vi "DrawOverlayImage.vi"(0 "reference":refnum<class "PackageNode.lvclass">, 1 "graphics":refnum<class "Graphics.lvclass">, 5 "error in (no error)":errorcluster) -> (14 "reference out":refnum<class "PackageNode.lvclass">, 15 "HotSpots":T1[](array[typedef]) {"HotSpot"."y" format="%.2f"; "HotSpot"."x" format="%.2f"}, 19 "error out":errorcluster)   [LabVIEW 2020, in "PackageNode.lvclass"]
doc: "Abstract draw"
uses:
  <resource>/Framework/Providers/Open_GDS/UML/PackageNode_class/PackageNode.lvclass
  C:/Program Files (x86)/National Instruments/LabVIEW 2020/resource/Framework/Providers/Open_GDS/UML/RectangularNode_class/RectangularNode.lvclass
  C:/Program Files (x86)/National Instruments/LabVIEW 2020/resource/Framework/Providers/Open_GDS/UML/AbstractNode_class/AbstractNode.lvclass
  <resource>/Framework/Providers/Open_GDS/UML/Graphics_class/Graphics.lvclass
  <resource>/Framework/Providers/Open_GDS/UML/UMLEditor/UMLEditor_HotSpotData.ctl
  <resource>/Framework/Providers/Open_GDS/UML/AbstractNode_class/AbstractNode.lvclass
  <resource>/Framework/Providers/Open_GDS/UML/General/Point/Point Point2D.ctl
  <resource>/Framework/Providers/Open_GDS/UML/UMLEditor/UMLEditor_HotSpotType.ctl
  <vilib>/picture/picture.llb/imagedata.ctl
  <resource>/Framework/Providers/Open_GDS/UML/RectangularNode_class/RectangularNode.lvclass
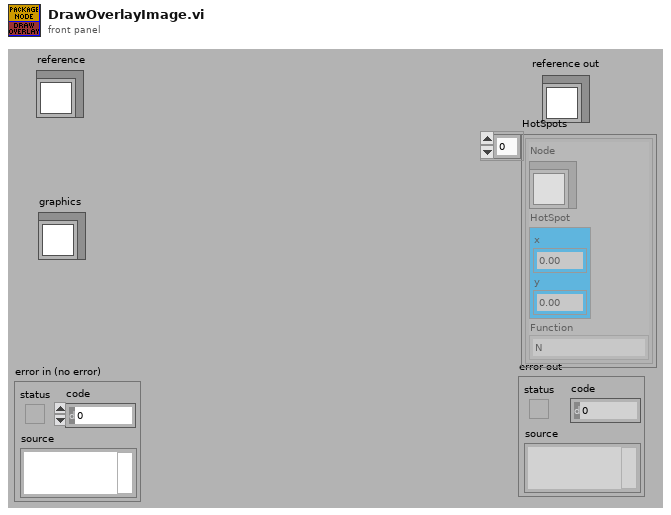
[diagram p1: front panel]
types:
  T1 = typedef "UMLEditor_HotSpotData.ctl" = cluster{"Node":refnum<class "AbstractNode.lvclass">, "HotSpot":T2, "Function":T3}
  T2 = typedef "Point Point2D.ctl" = cluster{"x":dbl, "y":dbl}
  T3 = typedef "UMLEditor_HotSpotType.ctl" = enum16{"N", "NE", "E", "SE", "S", "SW", "W", "NW", "Expand", "Collaps"}
  T4 = typedef "imagedata.ctl" = cluster{"image type":i32, "image depth":i32, "image":u8[], "mask":u8[], "colors":u32[], "Rectangle":cluster{"left":i16, "top":i16, "right":i16, "bottom":i16}}
  T5 = typedef "PackageNode.lvclass/ObjectAttributes.ctl" = cluster{"name":string, "contents":refnum<class "MultiLineString.lvclass">, "DEFAULT_TOP_WIDTH":i32, "DEFAULT_TOP_HEIGHT":i32, "DEFAULT_WIDTH":i32, "DEFAULT_HEIGHT":i32, "NAME_GAP":i32, "XGAP":i32, "YGAP":i32, "Collapsed":bool, "Note color":u32, "Justification":u16}
  T6 = typedef "RectangularNode.lvclass/ObjectAttributes.ctl" = cluster{"bounds":T7}
  T7 = typedef "Rectangle Rectangle2D.ctl" = cluster{"x":dbl, "y":dbl, "width":dbl, "height":dbl}
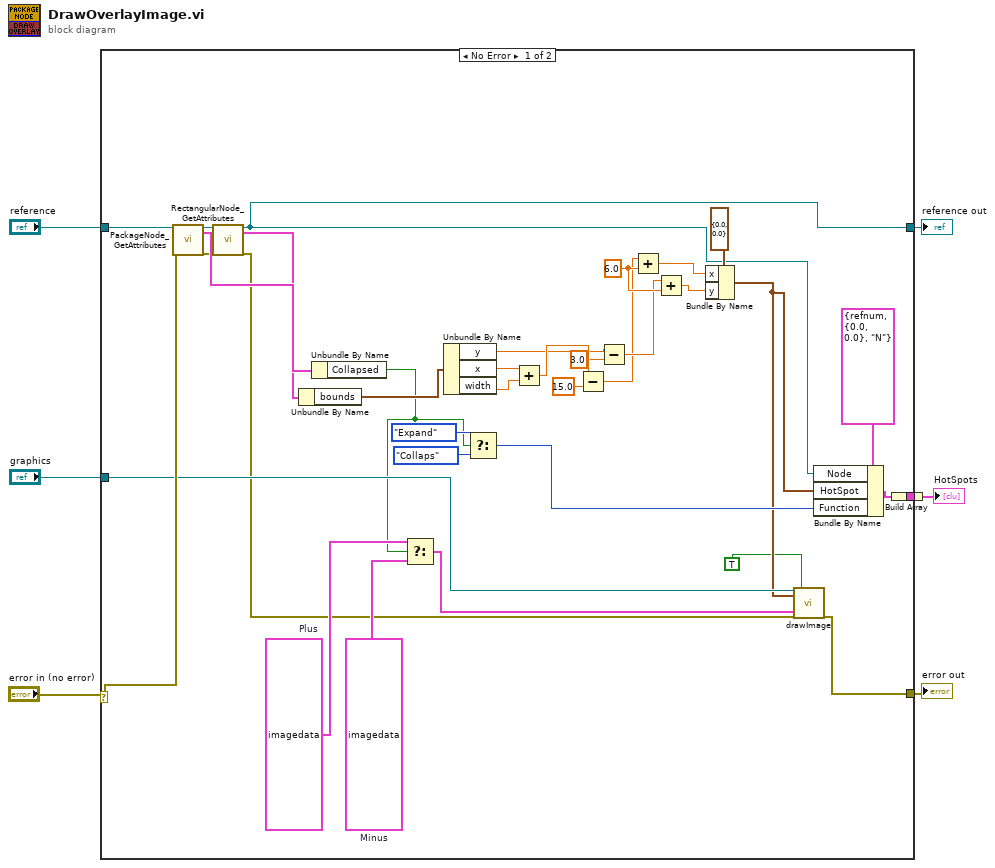
[diagram p0: block diagram]
diagram:
  n1 = case shown="No Error" "error in (no error)" {
    selector: "error in (no error)" -> [w40 w42]
    tunnel: "reference" -> [w41 w43]
    tunnel: [w39 w42] -> w5
    tunnel: [w8 w43] -> w4
    tunnel: "graphics" -> [w31 _]
    tunnel: [w25 _] -> w1
    frame No Error {
      w22 = 6.0 ("y")
      w29 = T4 {"image type"=0, "image depth"=24, "image"=[255, 255, 255, 255, 255, 255, 219, 227, 245, 189, 201, 232, 163, 178, 221, 155, 173, 221, 154, 171, 218, 154, 169, 213, 219, 227, 245, 255, 255, 255, 255, 255, 255, 255, 255, 255, 209, 218, 240, 167, 181, 222, 160, 175, 215, 178, 211, 235, 193, 242, 254, 184, 224, 246, 158, 184, 227, 158, 174, 219, 204, 213, 238, 255, 255, 255, 219, 227, 245, 168, 182, 223, 191, 204, 229, 255, 255, 255, 224, 247, 255, 183, 231, 255, 179, 229, 255, 190, 241, 255, 168, 212, 245, 156, 171, 218, 219, 227, 245, 192, 204, 235, 167, 186, 225, 239, 253, 255, 246, 252, 255, 196, 230, 255, 188, 238, 255, 176, 226, 255, 177, 228, 255, 198, 246, 255, 157, 186, 228, 169, 180, 218, 167, 183, 224, 178, 206, 236, 202, 245, 255, 177, 221, 249, 205, 254, 255, 205, 254, 255, 205, 254, 255, 205, 254, 255, 205, 254, 255, 188, 231, 249, 154, 171, 218, 157, 175, 222, 178, 216, 242, 180, 231, 255, 129, 179, 230, 1, 103, 204, 1, 103, 204, 1, 103, 204, 1, 103, 204, 221, 255, 255, 205, 252, 254, 155, 173, 221, 167, 182, 224, 176, 206, 238, 187, 238, 255, 194, 209, 227, 194, 209, 227, 194, 209, 227, 194, 209, 227, 194, 209, 227, 232, 255, 255, 201, 240, 249, 154, 171, 218, 192, 204, 235, 160, 179, 223, 197, 241, 255, 180, 230, 255, 207, 255, 255, 223, 255, 255, 242, 255, 255, 253, 255, 255, 250, 255, 255, 182, 209, 234, 169, 180, 218, 219, 227, 245, 161, 175, 218, 163, 198, 240, 199, 245, 255, 201, 251, 255, 218, 255, 255, 230, 255, 255, 241, 255, 255, 238, 242, 250, 159, 175, 219, 213, 220, 240, 255, 255, 255, 219, 227, 245, 155, 169, 212, 153, 179, 223, 187, 226, 249, 208, 251, 254, 201, 240, 249, 184, 211, 235, 159, 175, 219, 194, 202, 230, 255, 255, 255, 255, 255, 255, 255, 255, 255, 219, 227, 245, 185, 197, 230, 158, 173, 219, 155, 173, 221, 154, 171, 218, 176, 186, 225, 219, 227, 245, 255, 255, 255, 255, 255, 255], "mask"=[], "colors"=[], "Rectangle"={"left"=0, "top"=0, "right"=11, "bottom"=11}}  # Minus
      w30 = T4 {"image type"=0, "image depth"=24, "image"=[255, 255, 255, 255, 255, 255, 219, 227, 245, 172, 183, 221, 154, 171, 218, 155, 173, 221, 158, 174, 218, 173, 184, 223, 214, 222, 241, 255, 255, 255, 255, 255, 255, 255, 255, 255, 205, 214, 239, 158, 173, 218, 187, 206, 234, 197, 233, 249, 190, 240, 254, 184, 229, 249, 163, 196, 235, 156, 173, 220, 204, 213, 238, 255, 255, 255, 219, 227, 245, 154, 171, 217, 222, 234, 246, 255, 255, 255, 201, 235, 255, 184, 232, 255, 175, 226, 255, 190, 241, 255, 172, 218, 250, 154, 170, 217, 219, 227, 245, 186, 196, 231, 167, 193, 228, 229, 253, 255, 216, 238, 255, 145, 209, 244, 45, 116, 197, 199, 249, 255, 192, 242, 255, 198, 248, 255, 160, 187, 226, 174, 185, 222, 164, 179, 223, 185, 228, 246, 190, 235, 255, 145, 209, 244, 145, 209, 244, 45, 116, 197, 169, 221, 244, 191, 238, 250, 206, 255, 255, 190, 231, 249, 154, 171, 218, 157, 174, 222, 191, 241, 254, 174, 225, 255, 1, 103, 204, 45, 116, 197, 45, 116, 197, 45, 116, 197, 45, 116, 197, 218, 255, 255, 209, 253, 254, 155, 173, 221, 166, 181, 224, 178, 211, 241, 185, 236, 255, 155, 205, 242, 158, 208, 241, 45, 116, 197, 205, 220, 234, 205, 220, 234, 231, 255, 255, 196, 232, 244, 159, 175, 219, 190, 202, 233, 154, 173, 221, 198, 243, 255, 182, 232, 255, 183, 230, 242, 45, 116, 197, 248, 255, 255, 254, 255, 255, 253, 255, 255, 162, 183, 217, 184, 197, 229, 214, 222, 241, 156, 170, 210, 153, 181, 228, 192, 240, 255, 209, 255, 255, 216, 255, 255, 224, 255, 255, 238, 255, 255, 208, 221, 236, 162, 177, 220, 219, 227, 245, 255, 255, 255, 214, 222, 241, 161, 175, 216, 154, 173, 216, 159, 189, 224, 189, 221, 237, 190, 219, 237, 166, 182, 219, 164, 177, 220, 209, 218, 240, 255, 255, 255, 255, 255, 255, 255, 255, 255, 214, 222, 241, 192, 204, 235, 165, 179, 221, 157, 175, 222, 167, 182, 224, 192, 204, 235, 219, 227, 245, 255, 255, 255, 255, 255, 255], "mask"=[], "colors"=[], "Rectangle"={"left"=0, "top"=0, "right"=11, "bottom"=11}}  # Plus
      n2 = call <resource>:"PackageNode_GetAttributes.vi"("reference in"=w41, "error in (no error)"=w40) -> ("reference out"=w11:refnum<class "PackageNode.lvclass">, "Data"=w12:T5, "error out"=w10:errorcluster)  [unwired: 14 in, 1 out]
      n3 = call <resource>:"RectangularNode_GetAttributes.vi"("reference in"=w11, "error in (no error)"=w10) -> ("reference out"=w8:refnum<class "PackageNode.lvclass">, "Data"=w7:T6, "error out"=w9:errorcluster)  [unwired: 14 in, 1 out]
      n4 = Unbundle By Name(w7) -> ("bounds"=w38:T7)
      n5 = Unbundle By Name(w12) -> ("Collapsed"=w20:bool)
      n6 = Select(t=w30, s=w20, f=w29) -> (s? t:f=w28:T4)
      n7 = Unbundle By Name(w38) -> ("y"=w33:dbl, "x"=w37:dbl, "width"=w36:dbl)
      n8 = Select(t=UMLEditor_HotSpotType."Expand" ("Positions"), s=w20, f=UMLEditor_HotSpotType."Collaps" ("Positions")) -> (s? t:f=w19:T3)
      n9 = Add(x=w37, y=w36) -> (x+y=w35:dbl)
      n10 = Subtract(x=w35, y=15.0) -> (x-y=w17:dbl)
      n11 = Subtract(x=w33, y=3.0) -> (x-y=w18:dbl)
      n12 = Add(x=w17, y=w22) -> (x+y=w16:dbl)
      n13 = Add(x=w18, y=w22) -> (x+y=w15:dbl)
      n14 = Bundle By Name(cluster=T2 {"x"=0.0, "y"=0.0} ("HotSpot"), "x"=w16, "y"=w15) -> (w14:T2)
      n15 = call <resource>:"drawImage.vi"("reference"=w31, "Point"=w14, "Image"=w28, "error in (no error)"=w9, "PointInCenter(UpperRightCorner=F)"=TRUE) -> ("error out"=w39:errorcluster)  [unwired: 13 in, 1 out]
      n16 = Bundle By Name(cluster=T1 {"Node"=refnum, "HotSpot"={"x"=0.0, "y"=0.0}, "Function"=enum."N"} ("ObjectHotSpot"), "Node"=w8, "HotSpot"=w14, "Function"=w19) -> (w26:T1)
      n17 = Build Array(w26) -> (w25:T1[])
    }
    frame Error {
    }
  }
  "reference out" <- w4
  "error out" <- w5
  "HotSpots" <- w1
